vi "Build GetType.vi"(8 "error in (no error)":errorcluster, 10 "Get Type VI":refnum<vi>, 11 "CS++Actor in":refnum<class "CS++Actor.lvclass">) -> (0 "error out":errorcluster, 3 "CS++Actor out":refnum<class "CS++Actor.lvclass">)   [LabVIEW 2016, in "CS++Actor.lvlib" / "CS++Actor.lvclass"]
uses:
  CS++Actor.lvclass
  CS++Actor.lvclass/CS++Actor.ctl
  <vilib>/Utility/traverseref.llb/TRef TravTarget.ctl
  <vilib>/Utility/traverseref.llb/VI Scripting - Traverse.lvlib
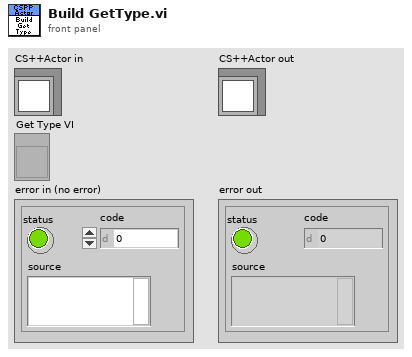
[diagram p1: front panel]
types:
  T1 = enum16{"Replace Class Controls/Indicator", "Connect Unbundler & Bundler"}
  T2 = enum16{"Invalid Wire Rule", "Required", "Recommended", "Optional", "Dynamic Dispatch"}
  T3 = typedef "TRef TravTarget.ctl" = enum16{"FP", "BD", "Other"}
  T4 = typedef "LVRectTypeDef.ctl" = cluster{"Left":i16, "Top":i16, "Right":i16, "Bottom":i16}
  T5 = enum16{"Invalid Wire Rule", "Required", "Recommended", "Optional", "Dynamic Dispatch"}[]
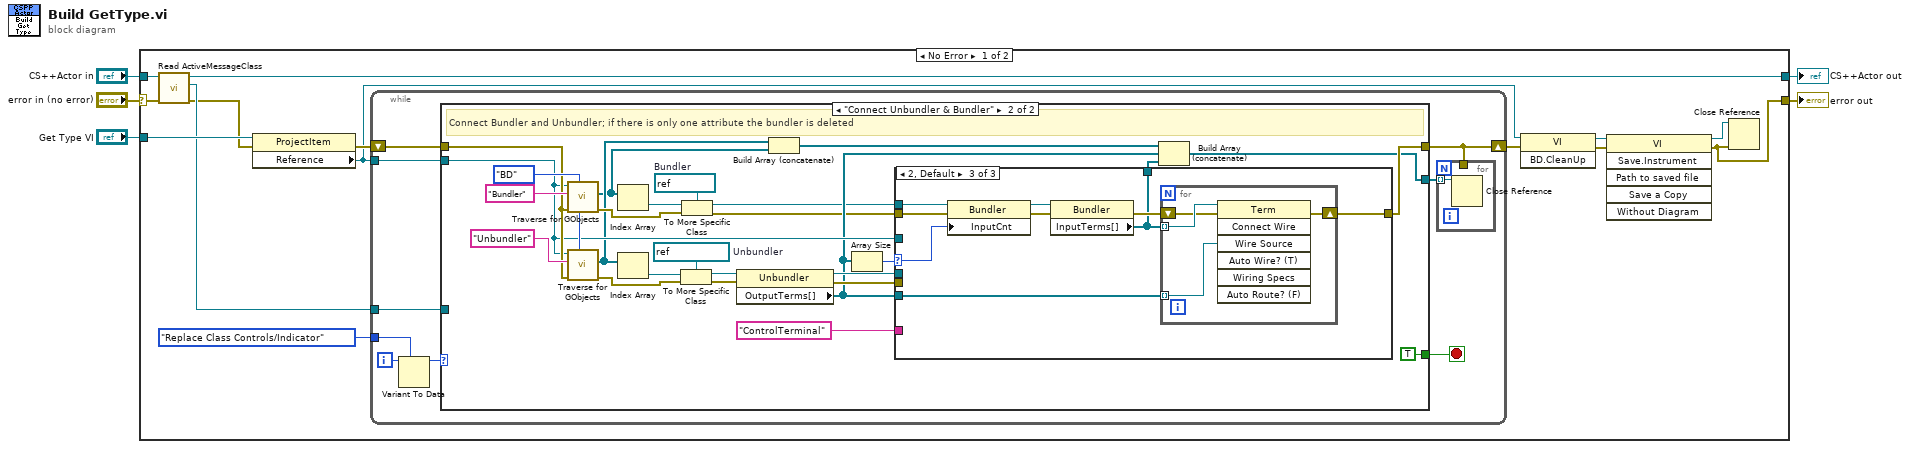
[diagram p0: block diagram]
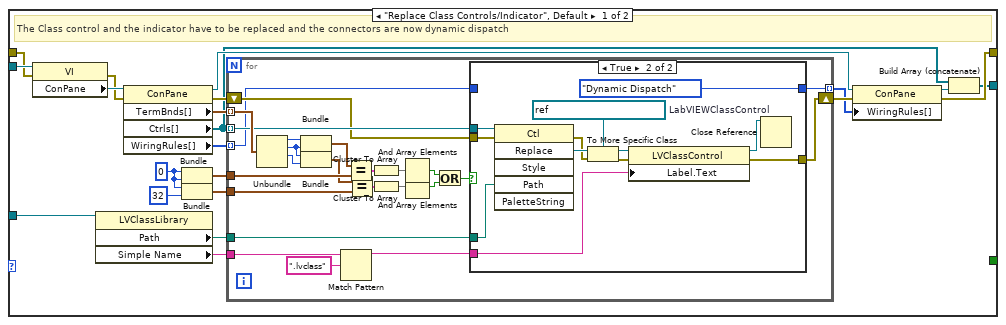
[diagram p2: hidden frame]
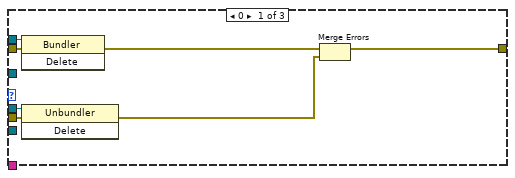
[diagram p4: hidden frame]
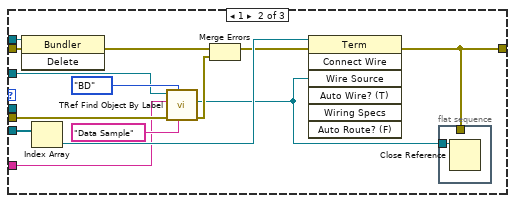
[diagram p5: hidden frame]
diagram:
  n1 = case shown="No Error" "error in (no error)" {
    selector: "error in (no error)" -> [w6 w152]
    tunnel: [w12 w152] -> w4
    tunnel: [w8 w151] -> w2
    tunnel: "CS++Actor in" -> [w7 w151]
    tunnel: "Get Type VI" -> [w18 _]
    frame No Error {
      n2 = call "Read ActiveMessageClass.vi"("error in (no error)"=w6, "CS++Actor in"=w7) -> ("error out"=w9:errorcluster, "ActiveMessageClass"=w10:refnum<vi>, "CS++Actor out"=w8:refnum<class "CS++Actor.lvclass">)  [unwired: 7 in]
      n3 = property class="ProjectItem"(reference=w18, error in=w9) -> (error out=w17:errorcluster, "Reference"=w13:refnum<vi>)  [unwired: 1 out]
      n4 = while {
        tunnel: T1."Replace Class Controls/Indicator" -> [w27]
        tunnel: w13 -> [w24]
        shift-right: [w20] -> w11
        shift-left: w17 -> [w25]
        tunnel: w10 -> [w23]
        i -> [w28]
        stop <- w22 stop-if-true
        n5 = Variant To Data(type=w27, Variant=w28) -> (data=w26:T1)  [unwired: 1 in, 1 out]
        n6 = case shown="\"Connect Unbundler & Bundler\"" w26 {
          tunnel: w25 -> [w49 w107]
          tunnel: w24 -> [w50 w99]
          tunnel: w23 -> [w41 _]
          tunnel: [w36 w98] -> w20
          tunnel: [_ TRUE] -> w22
          tunnel: [w31 w97] -> w21
          frame "Replace Class Controls/Indicator", Default {
            w39 = i16 0
            # "The Class control and the indicator have to be replaced and the connectors are now dynamic dispatch"
            n7 = property class="VI"(reference=w50, error in=w49) -> (error out=w47:errorcluster, "ConPane"=w48:refnum<vi>)  [unwired: 1 out]
            n8 = property class="LVClassLibrary"(reference=w41) -> ("Path"=w40:path, "Simple Name"=w30:string)  [unwired: 1 in, 2 out]
            n9 = property class="ConPane"(reference=w48, error in=w47) -> (reference out=w35:refnum<vi>, error out=w45:errorcluster, "TermBnds[]"=w46:T4[], "Ctrls[]"=w33:refnum<vi>[], "WiringRules[]"=w38:T5)
            n10 = Bundle(w39, w39) -> (w43:cluster{i16, i16})  [unwired: 1 in]
            n11 = Bundle(w39, i16 32) -> (w42:cluster{i16, i16})  [unwired: 1 in]
            n12 = for {
              tunnel: w46 -> [w74] mode=indexing
              tunnel: w33 -> [w64] mode=indexing
              shift-right: [w58] -> w37
              shift-left: w45 -> [w63]
              tunnel: w43 -> [w71]
              tunnel: w42 -> [w69]
              tunnel: w40 -> [w59]
              tunnel: w38 -> [w55] mode=indexing
              tunnel: [w54] -> w34 mode=indexing
              tunnel: w30 -> [w53]
              n13 = Unbundle(w74) -> ("Left"=w73:i16, "Top"=w56:i16, "Right"=w57:i16)  [unwired: 1 out]
              n14 = Bundle("Left"=w73, "Top"=w56) -> (w72:cluster{"Left":i16, "Top":i16})  [unwired: 1 in]
              n15 = Bundle("Top"=w56, "Right"=w57) -> (w70:cluster{"Top":i16, "Right":i16})  [unwired: 1 in]
              n16 = Match Pattern(string=w53, regular expression=".lvclass") -> (before substring=w52:string)  [unwired: 1 in, 3 out]
              n17 = Equal?(x=w72, y=w71) -> (x = y?=w68:cluster{bool, bool})
              n18 = Equal?(x=w70, y=w69) -> (x = y?=w67:cluster{bool, bool})
              n19 = Cluster To Array(cluster=w68) -> (array=w66:bool[])
              n20 = Cluster To Array(cluster=w67) -> (array=w65:bool[])
              n21 = And Array Elements(Boolean array=w66) -> (logical AND=w62:bool)
              n22 = And Array Elements(Boolean array=w65) -> (logical AND=w61:bool)
              n23 = Or(x=w62, y=w61) -> (x .or. y?=w60:bool)
              n24 = case shown="True" w60 {
                tunnel: w64 -> [_ w88]
                tunnel: w63 -> [w76 w87]
                tunnel: [w76 w79] -> w58
                tunnel: w59 -> [_ w86]
                tunnel: w55 -> [w75 _]
                tunnel: [w75 T2."Dynamic Dispatch" ("Wire Rule")] -> w54
                tunnel: w52 -> [_ w77]
                frame False {
                }
                frame True {
                  w84 = refnum<vi> refnum  # LabVIEWClassControl
                  n25 = invoke class="Ctl" method="Replace"(reference=w88, error in=w87, "Path"=w86) -> (error out=w80:errorcluster, "Replace"=w83:refnum<vi>)  [unwired: 3 in, 4 out]
                  n26 = To More Specific Class(target class=w84, reference=w83, error in=w80) -> (specific class reference=w82:refnum<vi>, error out=w81:errorcluster)
                  n27 = property class="LVClassControl"(reference=w82, error in=w81, "Label.Text"=w77) -> (reference out=w78:refnum<vi>, error out=w79:errorcluster)
                  n28 = Close Reference(reference=w78) -> ()  [unwired: 1 in, 1 out]
                }
              }
            }
            n29 = property class="ConPane"(reference=w35, error in=w37, "WiringRules[]"=w34) -> (reference out=w32:refnum<vi>, error out=w36:errorcluster)
            n30 = Build Array (concatenate)(w33, w32) -> (w31:refnum<vi>[])
          }
          frame "Connect Unbundler & Bundler" {
            w108 = TRef_TravTarget."BD" ("Traverse Target")
            w113 = refnum<vi> refnum  # Unbundler
            w114 = refnum<vi> refnum  # Bundler
            # "Connect Bundler and Unbundler; if there is only one attribute the bundler is deleted"
            n31 = call <vilib>:"Traverse for GObjects.vi"("Traverse Target"=w108, "error in (no error)"=w107, "Class Name"="Bundler", "VI Refnum"=w99) -> ("error out"=w106:errorcluster, "References"=w95:refnum<vi>[])  [unwired: 4 in, 2 out]
            n32 = call <vilib>:"Traverse for GObjects.vi"("Traverse Target"=w108, "error in (no error)"=w107, "Class Name"="Unbundler", "VI Refnum"=w99) -> ("error out"=w104:errorcluster, "References"=w96:refnum<vi>[])  [unwired: 4 in, 2 out]
            n33 = Index Array(array=w95) -> (element=w105:refnum<vi>)  [unwired: 1 in]
            n34 = Index Array(array=w96) -> (element=w103:refnum<vi>)  [unwired: 1 in]
            n35 = To More Specific Class(target class=w113, reference=w103, error in=w104) -> (specific class reference=w112:refnum<vi>, error out=w111:errorcluster)
            n36 = To More Specific Class(target class=w114, reference=w105, error in=w106) -> (specific class reference=w90:refnum<vi>, error out=w89:errorcluster)
            n37 = property class="Unbundler"(reference=w112, error in=w111) -> (reference out=w100:refnum<vi>, error out=w102:errorcluster, "OutputTerms[]"=w92:refnum<vi>[])
            n38 = Build Array (concatenate)(w96, w95) -> (w94:refnum<vi>[])
            n39 = Array Size(array=w92) -> (size(s)=w101:i32)
            n40 = case shown="2, Default" w101 {
              selector: w101 -> [_ _ w143]
              tunnel: w90 -> [w122 w136 w144]
              tunnel: w89 -> [w121 w135 w145]
              tunnel: w102 -> [w119 w134 _]
              tunnel: w100 -> [w120 _ _]
              tunnel: w92 -> [_ w131 w146]
              tunnel: w99 -> [_ w129 _]
              tunnel: [w118 w124 w142] -> w98
              tunnel: "ControlTerminal" ("Class Name") -> [_ w123 _]
              tunnel: [_ _ w138] -> w91
              frame 0 {
                n41 = invoke class="Bundler" method="Delete"(reference=w122, error in=w121) -> (error out=w117:errorcluster)  [unwired: 1 in, 2 out]
                n42 = invoke class="Unbundler" method="Delete"(reference=w120, error in=w119) -> (error out=w116:errorcluster)  [unwired: 1 in, 2 out]
                n43 = Merge Errors(w117, w116) -> (w118:errorcluster)
              }
              frame 1 {
                n44 = invoke class="Bundler" method="Delete"(reference=w136, error in=w135) -> (error out=w128:errorcluster)  [unwired: 1 in, 2 out]
                n45 = Index Array(array=w131) -> (element=w130:refnum<vi>)  [unwired: 1 in]
                n46 = call <vilib>:"TRef Find Object By Label.vi"("Label"="Data Sample", "Traverse Target"=TRef_TravTarget."BD", "error in (no error)"=w134, "Class Name"=w123, "VI Ref"=w129) -> ("error out"=w127:errorcluster, "Found Obj Ref"=w125:refnum<vi>)  [unwired: 3 in, 2 out]
                n47 = Merge Errors(w128, w127) -> (w126:errorcluster)
                n48 = invoke class="Term" method="Connect Wire"(reference=w130, error in=w126, "Wire Source"=w125) -> (error out=w124:errorcluster)  [unwired: 4 in, 6 out]
                n49 = flat-sequence {
                  tunnel: w125 -> [w137]
                  tunnel: w124 -> [_]
                  frame #0 {
                    n50 = Close Reference(reference=w137) -> ()  [unwired: 1 in, 1 out]
                  }
                }
              }
              frame 2, Default {
                n51 = property class="Bundler"(reference=w144, error in=w145, "InputCnt"=w143) -> (reference out=w141:refnum<vi>, error out=w140:errorcluster)
                n52 = property class="Bundler"(reference=w141, error in=w140) -> (error out=w139:errorcluster, "InputTerms[]"=w138:refnum<vi>[])  [unwired: 1 out]
                n53 = for {
                  tunnel: w146 -> [w147] mode=indexing
                  shift-right: [w148] -> w142
                  shift-left: w139 -> [w149]
                  tunnel: w138 -> [w150] mode=indexing
                  n54 = invoke class="Term" method="Connect Wire"(reference=w150, error in=w149, "Wire Source"=w147) -> (error out=w148:errorcluster)  [unwired: 4 in, 6 out]
                }
              }
            }
            n55 = Build Array (concatenate)(w94, w92, w91) -> (w97:refnum<vi>[])
          }
        }
        n56 = for {
          tunnel: w21 -> [w29] mode=indexing
          tunnel: w20 -> [_]
          n57 = Close Reference(reference=w29) -> ()  [unwired: 1 in, 1 out]
        }
      }
      n58 = invoke class="VI" method="BD.CleanUp"(reference=w13, error in=w11) -> (reference out=w16:refnum<vi>, error out=w14:errorcluster)  [unwired: 1 in, 1 out]
      n59 = invoke class="VI" method="Save.Instrument"(reference=w16, error in=w14) -> (reference out=w15:refnum<vi>, error out=w12:errorcluster)  [unwired: 4 in, 4 out]
      n60 = Close Reference(reference=w15, error in (no error)=w12) -> ()  [unwired: 1 out]
    }
    frame Error {
    }
  }
  "error out" <- w4
  "CS++Actor out" <- w2
